vi "Result.Attribute Look Up Result Code.vi"(0 "Attribute":T1 {"Status" items=["LOG", "PASS", "FAIL", "ERROR"]}, 1 "error in":errorcluster, 4 "Limits":variant) -> (5 "Attribute":T1 {"Status" items=["LOG", "PASS", "FAIL", "ERROR"]})   [LabVIEW 2019]
uses:
  Result.Attribute.ctl
  Result.Measurement and Attribute Item Status.ctl
  Result.Test Limit Item.ctl
  Result.Limit Type.ctl
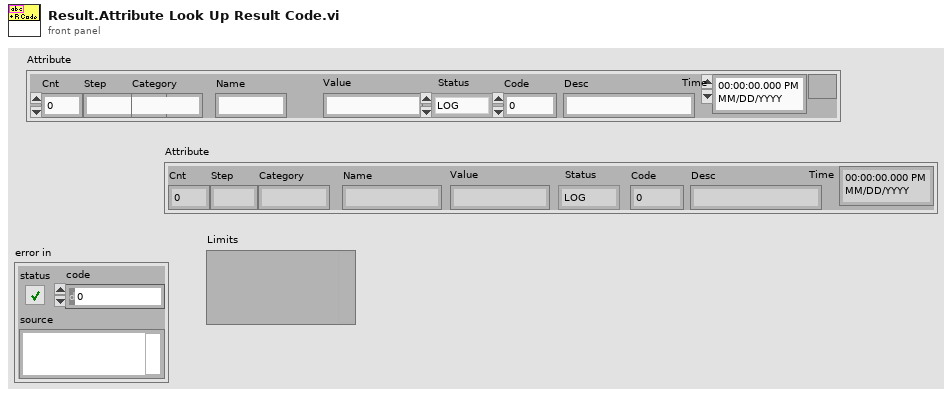
[diagram p1: front panel]
types:
  T1 = typedef "Result.Attribute.ctl" = cluster{"Cnt":i32, "Step":string, "Category":string, "Name":string, "Value":string, "Status":T2, "Code":i32, "Desc":string, "Time":timestamp}
  T2 = typedef "Result.Measurement and Attribute Item Status.ctl" = i32
  T3 = typedef "Result.Test Limit Item.ctl" = cluster{"Name":string, "LimType":T4, "LL":string, "UL":string, "Units":string, "FailCode":i32, "FailDesc":string}
  T4 = typedef "Result.Limit Type.ctl" = enum16{"None", "EQ", "NE", "GT", "LT", "GE", "LE", "GTLT", "GELE", "GELT", "GTLE", "LTGT", "LEGE", "LEGT", "LTGE", "Contains", "NotContains"}
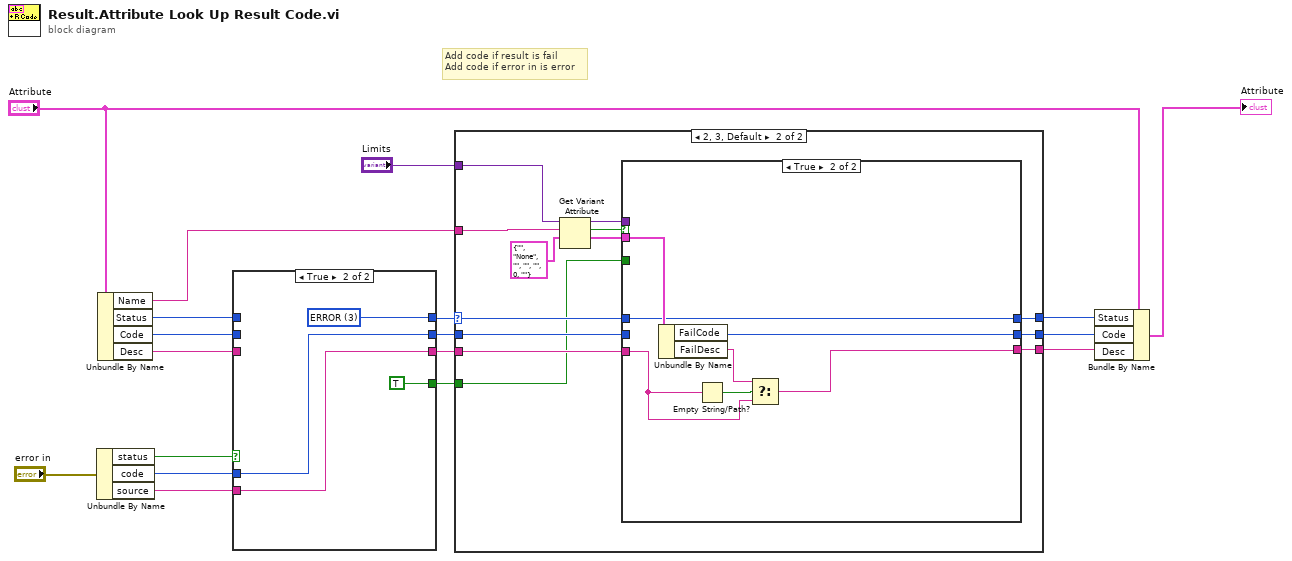
[diagram p0: block diagram]
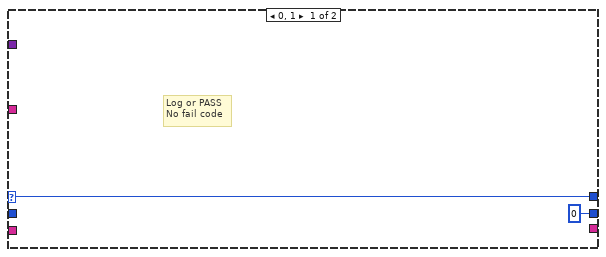
[diagram p2: hidden frame]
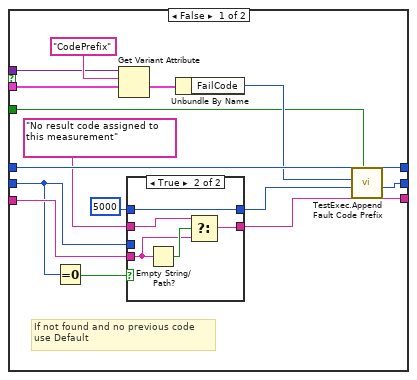
[diagram p3: hidden frame]
diagram:
  # "Add code if result is fail\nAdd code if error in is error"
  n1 = Unbundle By Name("error in") -> ("status"=w15:bool, "code"=w13:i32, "source"=w12:string)
  n2 = Unbundle By Name("Attribute") -> ("Name"=w6:string, "Status"=w14:T2, "Code"=w3:i32, "Desc"=w2:string)
  n3 = case shown="True" w15 {
    tunnel: [w21 w23] -> w11
    tunnel: w14 -> [w21 _]
    tunnel: w13 -> [_ w25]
    tunnel: [w20 w25] -> w9
    tunnel: w12 -> [_ w24]
    tunnel: [w19 w24] -> w8
    tunnel: w3 -> [w20 _]
    tunnel: w2 -> [w19 _]
    tunnel: [_ TRUE] -> w1
    frame False {
    }
    frame True {
      w23 = T2 3 items=["LOG", "PASS", "FAIL", "ERROR"] ("Status")
    }
  }
  n4 = case shown="2, 3, Default" w11 {
    selector: w11 -> [w27 w32]
    tunnel: [w27 w31] -> w10
    tunnel: w9 -> [_ w30]
    tunnel: w8 -> [_ w29]
    tunnel: [0 ("FailCode") w35] -> w7
    tunnel: w6 -> [_ w36]
    tunnel: [_ w34] -> w5
    tunnel: "Limits" -> [_ w33]
    tunnel: w1 -> [_ w28]
    frame 0, 1 {
      # "Log or PASS\nNo fail code"
    }
    frame 2, 3, Default {
      n5 = Get Variant Attribute(Variant=w33, name=w36, default value (empty Variant)=T3 {"Name"="", "LimType"=enum."None", "LL"="", "UL"="", "Units"="", "FailCode"=0, "FailDesc"=""} ("Result.Test Limit Item")) -> (duplicate Variant=w39:variant, found=w40:bool, value=w38:T3)  [unwired: 1 in, 1 out]
      n6 = case shown="True" w40 {
        tunnel: w39 -> [w46 _]
        tunnel: w38 -> [w45 w68]
        tunnel: [w44 w69] -> w35
        tunnel: [w51 w63] -> w34
        tunnel: w32 -> [w55 w67]
        tunnel: [w55 w67] -> w31
        tunnel: w30 -> [w52 _]
        tunnel: w29 -> [w53 w64]
        tunnel: w28 -> [w41 _]
        frame False {
          # "If not found and no previous code\nuse Default"
          n7 = Equal To 0?(x=w52) -> (x = 0?=w54:bool)
          n8 = Get Variant Attribute(Variant=w46, name="CodePrefix", default value (empty Variant)=w45) -> (value=w48:T3)  [unwired: 1 in, 3 out]
          n9 = case shown="True" w54 {
            tunnel: w53 -> [w56 w58]
            tunnel: w52 -> [w57 _]
            tunnel: 5000 ("Code") -> [_ w62]
            tunnel: "No result code assigned to this measurement" ("Desc") -> [_ w60]
            tunnel: [w57 w62] -> w43
            tunnel: [w56 w59] -> w51
            frame False {
            }
            frame True {
              n10 = Empty String/Path?(string/path=w58) -> (empty?=w61:bool)
              n11 = Select(t=w60, s=w61, f=w58) -> (s? t:f=w59:string)
            }
          }
          n12 = Unbundle By Name(w48) -> ("FailCode"=w42:i32)
          n13 = call "TestExec.Append Fault Code Prefix.vi"("Positive(F)\\Negative(T)"=w41, "FaultCode"=w43, "FaultCode Prefix"=w42) -> ("New Fault Code"=w44:i32)  [unwired: 8 in]
        }
        frame True {
          n14 = Unbundle By Name(w68) -> ("FailCode"=w69:i32, "FailDesc"=w65:string)
          n15 = Empty String/Path?(string/path=w64) -> (empty?=w66:bool)
          n16 = Select(t=w65, s=w66, f=w64) -> (s? t:f=w63:string)
        }
      }
    }
  }
  n17 = Bundle By Name(cluster="Attribute", "Status"=w10, "Code"=w7, "Desc"=w5) -> (→"Attribute":T1)
